vi "Init.vi"(8 "error in (no error)":errorcluster, 10 "VIEW":refnum<class "VIEW.lvclass">, 11 "MyAppController in":refnum<class "MyAppController.lvclass">) -> (0 "error out":errorcluster, 3 "MyAppController out":refnum<class "MyAppController.lvclass">)   [LabVIEW 2013, in "MyAppController.lvclass"]
uses:
  MyAppController.lvclass
  Framework/View/base/VIEW.lvclass
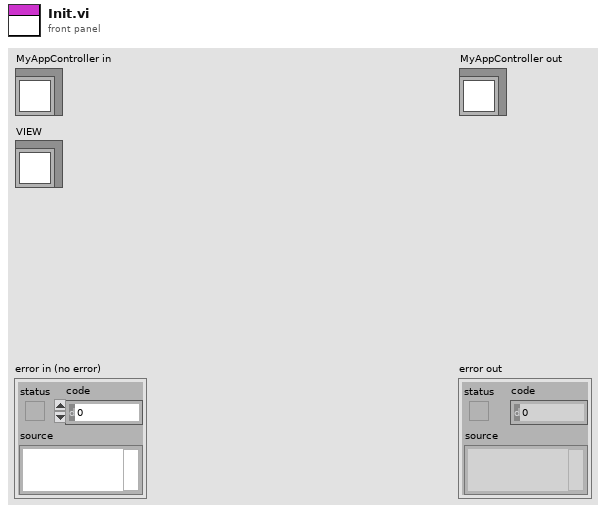
[diagram p1: front panel]
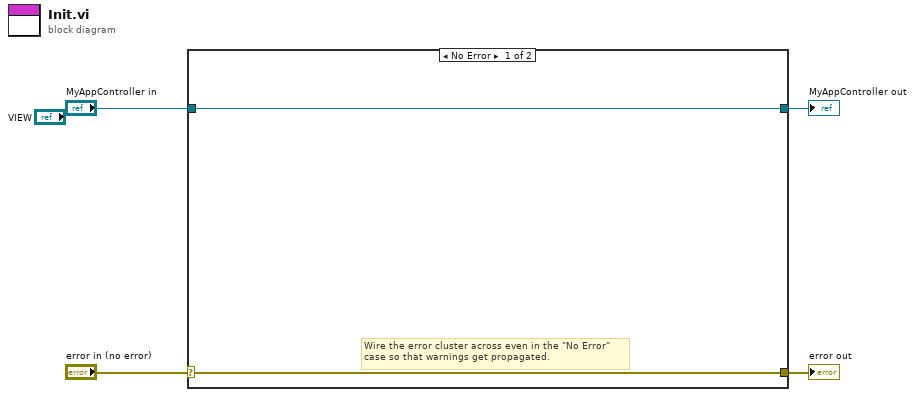
[diagram p0: block diagram]
diagram:
  n1 = case shown="No Error" "error in (no error)" {
    selector: "error in (no error)" -> [w5 w8]
    tunnel: [w5 w8] -> w3
    tunnel: [w6 w7] -> w1
    tunnel: "MyAppController in" -> [w6 w7]
    frame No Error {
      # "Wire the error cluster across even in the \"No Error\"\ncase so that warnings get propagated."
    }
    frame Error {
    }
  }
  "error out" <- w3
  "MyAppController out" <- w1
